vi "Example.vi"() -> ()   [LabVIEW 2022 SP3, in "FHPP.lvclass"]
uses:
  FHPP.lvclass
  TypeDefs/Operating Mode.ctl
  TypeDefs/DIR.ctl
  TypeDefs/CCON.ctl
  TypeDefs/Setpoints.ctl
  TypeDefs/CPOS.ctl
  FHPP.lvclass/FHPP.ctl
panel:
  in  "data value 4":T1
  in  "data value 3":T2 {"Setpoint" max=100; "Vel/VelRamp (%)" max=100}
  in  "data value 2":T3
  in  "data value":T5
  in  "stop":bool
  in  "Operating Mode 2":T4
  out "Operating Mode":T4
  out "error out 2":errorcluster
  out "error out":errorcluster
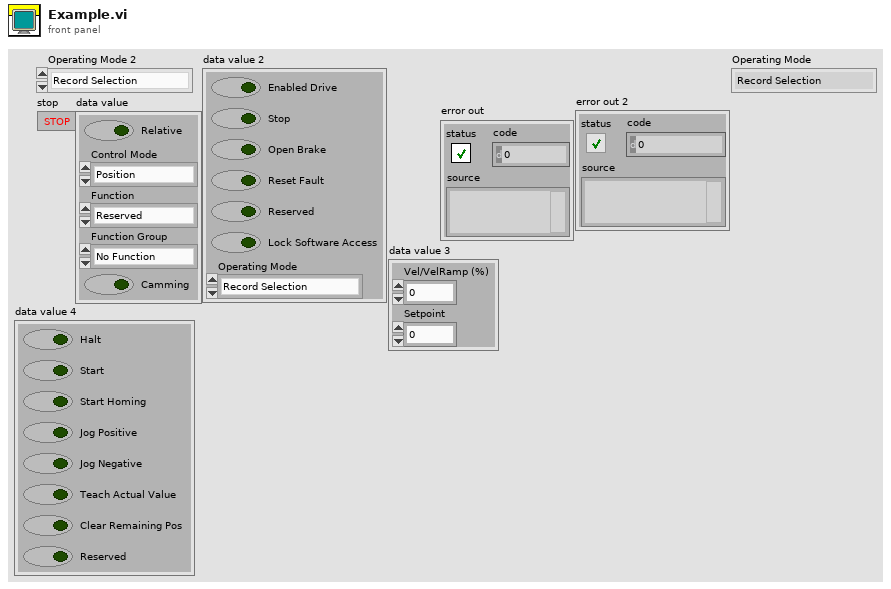
[diagram p1: front panel]
types:
  T1 = typedef "FHPP.lvclass/CPOS.ctl" = cluster{"Halt":bool, "Start":bool, "Start Homing":bool, "Jog Positive":bool, "Jog Negative":bool, "Teach Actual Value":bool, "Clear Remaining Pos":bool, "Reserved":bool}
  T2 = typedef "FHPP.lvclass/Setpoints.ctl" = cluster{"Vel/VelRamp (%)":u8, "Setpoint":u32}
  T3 = typedef "FHPP.lvclass/CCON.ctl" = cluster{"Enabled Drive":bool, "Stop":bool, "Open Brake":bool, "Reset Fault":bool, "Reserved":bool, "Lock Software Access":bool, "Operating Mode":T4}
  T4 = typedef "FHPP.lvclass/Operating Mode.ctl" = enum16{"Record Selection", "Direct Mode", "Reserved 1", "Reserved 2"}
  T5 = typedef "FHPP.lvclass/DIR.ctl" = cluster{"Relative":bool, "Control Mode":enum8{"Position", "Force", "Velocity", "Reserved"}, "Function":enum8{"Reserved", "External Input", "External Input with  Cam", "Virtual Master with Cam"}, "Function Group":enum8{"No Function", "Reserver 1", "Reserved 2", "Reserved 3"}, "Camming":bool}
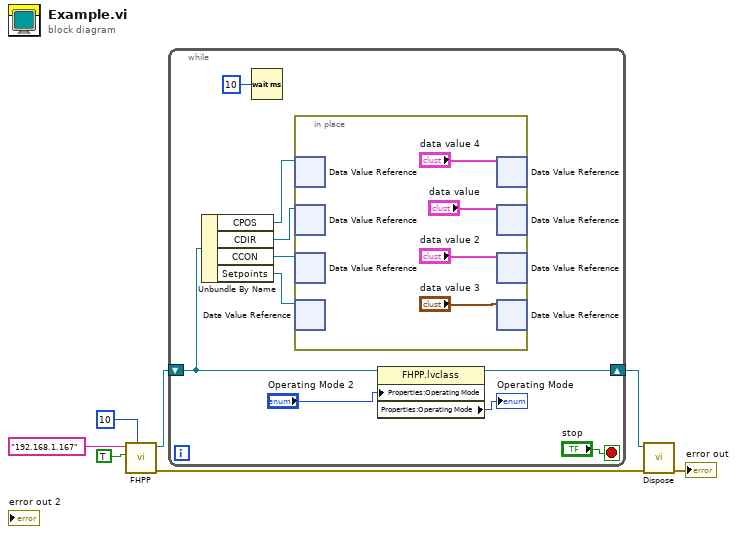
[diagram p0: block diagram]
diagram:
  n1 = call "FHPP.vi"("Cyle (ms)"=10, "Use FCT"=TRUE, "IP Address"="192.168.1.167") -> ("error out"=w4:errorcluster, "FHPP out"=w2:refnum<class "FHPP.lvclass">)  [unwired: 7 in]
  n2 = while {
    shift-right: [w17] -> w1
    shift-left: w2 -> [w12]
    stop <- "stop" stop-if-true
    n3 = Unbundle By Name(w12) -> ("CPOS"=w8:refnum<data-value>, "CDIR"=w11:refnum<data-value>, "CCON"=w10:refnum<data-value>, "Setpoints"=w9:refnum<data-value>)
    n4 = Wait (ms)(milliseconds to wait=u32 10) -> ()  [unwired: 1 out]
    n5 = in-place {
      n6 = in-place-dvr #1(w8) -> ()  [unwired: 2 out]
      n7 = in-place-dvr #2(w11) -> ()  [unwired: 2 out]
      n8 = in-place-dvr #3(w10) -> ()  [unwired: 2 out]
      n9 = in-place-dvr #4(w9) -> ()  [unwired: 2 out]
      n10 = in-place-dvr #1("data value 4") -> ()  [unwired: 2 out]
      n11 = in-place-dvr #2("data value") -> ()  [unwired: 2 out]
      n12 = in-place-dvr #3("data value 2") -> ()  [unwired: 2 out]
      n13 = in-place-dvr #4("data value 3") -> ()  [unwired: 2 out]
    }
    n14 = property class="FHPP.lvclass"(reference=w12, "Properties:Operating Mode"="Operating Mode 2") -> (reference out=w17:refnum<class "FHPP.lvclass">, "Properties:Operating Mode"=→"Operating Mode":T4)  [unwired: 1 in, 1 out]
  }
  n15 = call-dynamic "Dispose.vi"("error in (no error)"=w4, "FHPP in"=w1) -> ("error out"=→"error out":errorcluster)  [unwired: 9 in]
